vi "Configure Number of Frames.vi"(8 "error in (no error)":errorcluster, 10 "number of frames":u32, 11 "TroSpec in":refnum<class "PL ISTEQ TroSpec.lvclass">) -> (0 "error out":errorcluster, 3 "TroSpec out":refnum<class "PL ISTEQ TroSpec.lvclass">)   [LabVIEW 2015, in "PL ISTEQ TroSpec.lvclass"]
doc: "Configures number of frames."
uses:
  PL ISTEQ TroSpec.lvclass
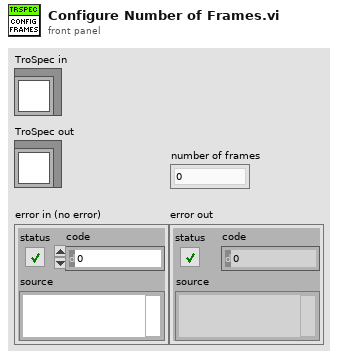
[diagram p1: front panel]
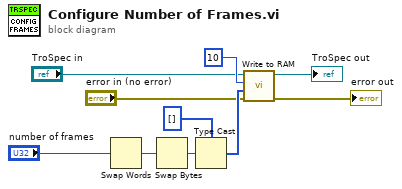
[diagram p0: block diagram]
diagram:
  n1 = Swap Words(1:"number of frames") -> (0:w1:u32)
  n2 = Swap Bytes(anything=w1) -> (byte swapped=w3:u32)
  n3 = Type Cast(type=u8[] [] ("data"), x=w3) -> (*(type *) &x=w10:u8[])
  n4 = call "Write to RAM.vi"("error in (no error)"="error in (no error)", "data"=w10, "address"=u16 10, "TroSpec in"="TroSpec in") -> ("error out"=→"error out":errorcluster, "TroSpec out"=→"TroSpec out":refnum<class "PL ISTEQ TroSpec.lvclass">)  [unwired: 6 in]
